vi "niTuner Set Freq(spec).vi"(8 "error in":errorcluster, 10 "desired RF spectrum settings":T3 {"resolution bandwidth" format="%.2p"; "RF frequency" format="%.2p"; "span" format="%.2p"}, 11 "taskID in":i32 format="%.0x") -> (0 "error out":errorcluster, 1 "RF tuned spectrum settings":T1 {"resolution bandwidth" format="%.2p"; "RF tuned frequency" format="%.2p"; "span" format="%.2p"}, 2 "actual IF spectrum settings":T2 {"resolution bandwidth" format="%.2p"; "IF frequency" format="%.2p"; "span" format="%.2p"}, 3 "taskID out":i32 format="%.0x", 4 "frequency shift":dbl format="%.2f")   [LabVIEW 2011]
doc: "This polymorph of Set Freq for SMT.vi sets a single spectrum and immediately begins to settle at the center frequency. The format of the \"spectrum settings\" inputs and outputs is designed to provide a convenient interface with the Spectral Measurements Toolset (SMT).\n\nNOTE: If new center frequencies of less than 15 MHz are specified by a call to this VI, attenuation may be automatically adjusted. Up to 20 dB additional attenuation may be added."
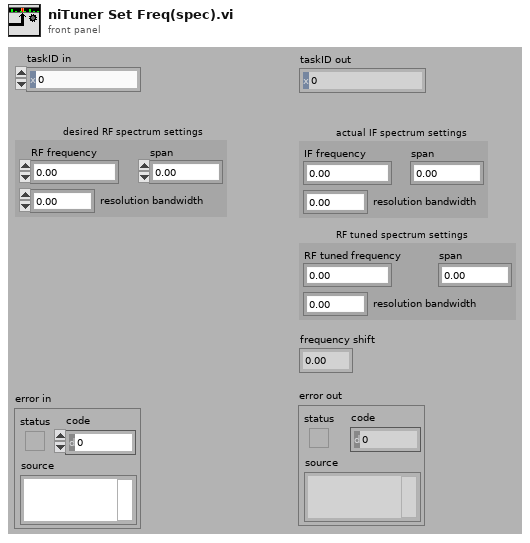
[diagram p1: front panel]
types:
  T1 = cluster{"RF tuned frequency":dbl, "span":dbl, "resolution bandwidth":dbl}
  T2 = cluster{"IF frequency":dbl, "span":dbl, "resolution bandwidth":dbl}
  T3 = cluster{"RF frequency":dbl, "span":dbl, "resolution bandwidth":dbl}
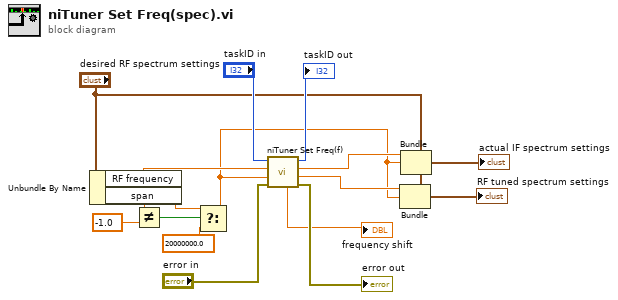
[diagram p0: block diagram]
diagram:
  n1 = Unbundle By Name("desired RF spectrum settings") -> ("RF frequency"=w10:dbl, "span"=w13:dbl)
  n2 = Not Equal?(x=w13, y=-1.0) -> (x != y?=w12:bool)
  n3 = Select(t=w13, s=w12, f=20000000.0) -> (s? t:f=w1:dbl)
  n4 = call <instrlib>:"niTuner Set Freq(f).vi"("error in"="error in", "span"=w1, "desired RF frequency"=w10, "taskID in"="taskID in") -> ("error out"=→"error out":errorcluster, "actual RF tuned frequency"=w5:dbl, "actual IF frequency"=w6:dbl, "taskID out"=→"taskID out":i32, "frequency shift"=→"frequency shift":dbl)  [unwired: 3 in]
  n5 = Bundle(cluster="desired RF spectrum settings", "RF frequency"=w5, "span"=w1) -> (→"RF tuned spectrum settings":T3)  [unwired: 1 in]
  n6 = Bundle(cluster="desired RF spectrum settings", "RF frequency"=w6, "span"=w1) -> (→"actual IF spectrum settings":T3)  [unwired: 1 in]
